vi "Calculate Cubic Bezier Points From Array.vi"(7 "t":dbl[](array[numeric]), 8 "d":dbl, 9 "c":dbl, 10 "b":dbl, 11 "a":dbl) -> (3 "f(t)":dbl[](array[numeric]))   [LabVIEW 2019, in "Tool Path.lvclass"]
uses:
  Tool Path.lvclass
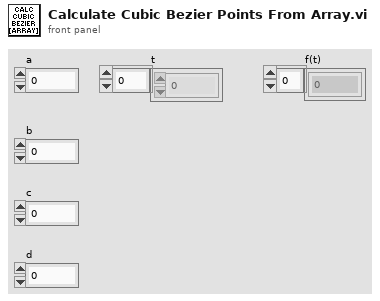
[diagram p1: front panel]
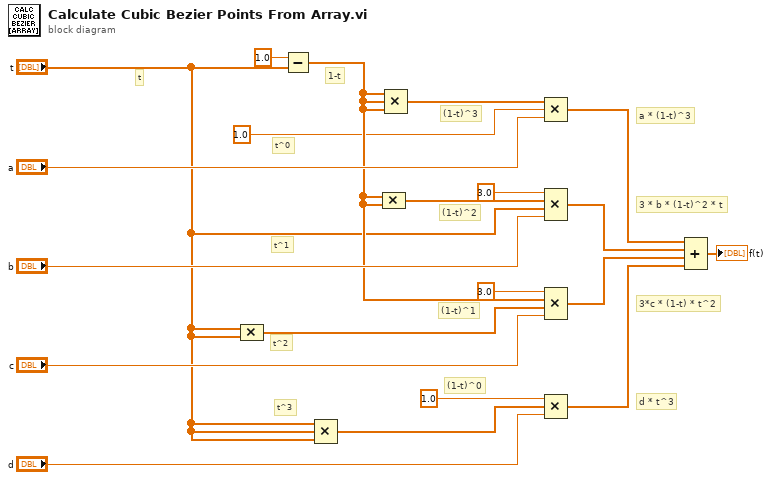
[diagram p0: block diagram]
diagram:
  # "(1-t)^0"
  # "t^3"
  # "t^2"
  # "t^1"
  # "t^0"
  # "(1-t)^1"
  # "(1-t)^2"
  # "(1-t)^3"
  # "1-t"
  # "d * t^3"
  # "3*c * (1-t) * t^2"
  # "3 * b * (1-t)^2 * t"
  # "a * (1-t)^3"
  # "t"
  n1 = Compound Arithmetic op=MULTIPLY("t", "t") -> (w3:dbl[])
  n2 = Subtract(x=1.0, y="t") -> (x-y=w6:dbl[])
  n3 = Compound Arithmetic op=MULTIPLY("t", "t", "t") -> (w4:dbl[])
  n4 = Compound Arithmetic op=MULTIPLY(w6, w6) -> (w8:dbl[])
  n5 = Compound Arithmetic op=MULTIPLY(w6, w6, w6) -> (w7:dbl[])
  n6 = Compound Arithmetic op=MULTIPLY(w7, 1.0, "a") -> (w13:dbl[])
  n7 = Compound Arithmetic op=MULTIPLY(3.0 ("value"), w8, "t", "b") -> (w12:dbl[])
  n8 = Compound Arithmetic op=MULTIPLY(3.0 ("value"), w6, w3, "c") -> (w11:dbl[])
  n9 = Compound Arithmetic op=MULTIPLY(1.0, w4, "d") -> (w10:dbl[])
  n10 = Compound Arithmetic op=ADD(w13, w12, w11, w10) -> (→"f(t)":dbl[])
